vi "Load Suite from Index.vi"(8 "error in (no error)":errorcluster, 11 "Path":path) -> (0 "error out":errorcluster, 3 "LUnit Test Suite out":refnum<class "LUnit Test Suite.lvclass">)   [LabVIEW 2020, in "Test Finder.lvclass"]
uses:
  Test Finder.lvclass
  LUnit Test Suite.lvclass
  C:/git/astemes-lunit/source/Runnable.lvclass
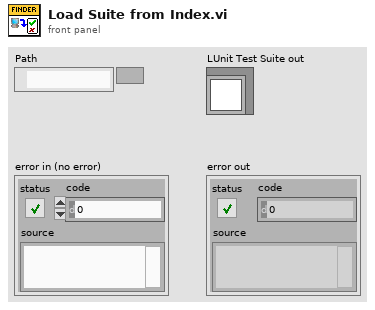
[diagram p1: front panel]
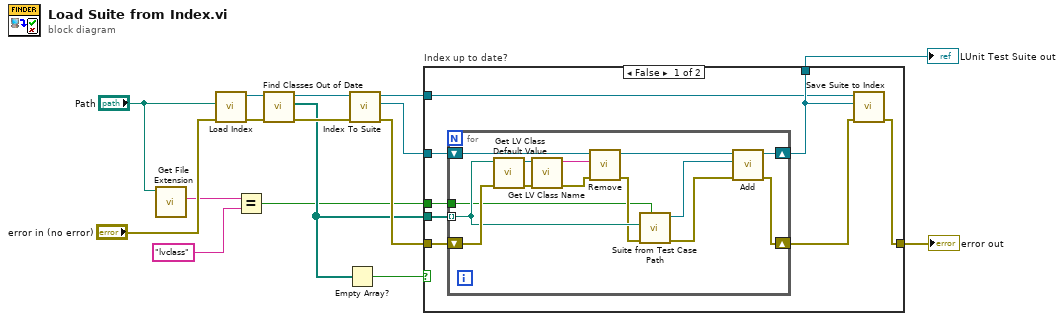
[diagram p0: block diagram]
diagram:
  n1 = call <vilib>:"Get File Extension.vi"("file"="Path") -> ("lowercase file extension"=w3:string)  [unwired: 6 in, 4 out]
  n2 = call "Load Index.vi"("error in (no error)"="error in (no error)", "Path"="Path") -> ("error out"=w9:errorcluster, "Test Finder out"=w8:refnum<class "Test Finder.lvclass">)  [unwired: 8 in]
  n3 = Equal?(x=w3, y="lvclass") -> (x = y?=w1:bool)
  n4 = call "Find Classes Out of Date.vi"("error in (no error)"=w9, "Test Finder In"=w8) -> ("error out"=w11:errorcluster, "Outdated Test Class paths"=w6:path[], "Test Finder Out"=w10:refnum<class "Test Finder.lvclass">)  [unwired: 7 in]
  n5 = Empty Array?(array=w6) -> (empty?=w5:bool)
  n6 = call "Index To Suite.vi"("error in (no error)"=w11, "Test Finder In"=w10) -> ("error out"=w12:errorcluster, "Suite"=w13:refnum<class "LUnit Test Suite.lvclass">, "Test Finder Out"=w14:refnum<class "Test Finder.lvclass">)  [unwired: 7 in]
  n7 = case "Index up to date?" shown="False" w5 {
    tunnel: [w24 w39] -> w16
    tunnel: [w23 w40] -> w15
    tunnel: w14 -> [w21 _]
    tunnel: w13 -> [w20 w40]
    tunnel: w12 -> [w19 w39]
    tunnel: w6 -> [w18 _]
    tunnel: w1 -> [w17 _]
    frame False {
      n8 = for {
        tunnel: w18 -> [w29] mode=indexing
        shift-right: [w37] -> w23
        shift-left: w20 -> [w38]
        shift-right: [w36] -> w22
        shift-left: w19 -> [w31]
        tunnel: w17 -> [w25]
        n9 = call <vilib>:"Get LV Class Default Value.vi"("error in (no error)"=w31, "class path"=w29) -> ("error out"=w34:errorcluster, "object"=w33:refnum<class>)  [unwired: 8 in]
        n10 = call <vilib>:"Get LV Class Name.vi"("error in (no error)"=w34, "object"=w33) -> ("error out"=w30:errorcluster, "class name"=w32:string)  [unwired: 8 in]
        n11 = call "Remove.vi"("error in (no error)"=w30, "Test to Remove"=w32, "LUnit Test Suite In"=w38) -> ("error out"=w28:errorcluster, "LUnit Test Suite Out"=w35:refnum<class "LUnit Test Suite.lvclass">)  [unwired: 7 in]
        n12 = call "Suite from Test Case Path.vi"("Ignore Index?"=w25, "error in (no error)"=w28, "Test Case"=w29) -> ("error out"=w26:errorcluster, "LUnit Test Suite Out"=w27:refnum<class "LUnit Test Suite.lvclass">)  [unwired: 7 in]
        n13 = call "Add.vi"("error in (no error)"=w26, "Runnable"=w27, "LUnit Test Suite In"=w35) -> ("error out"=w36:errorcluster, "LUnit Test Suite Out"=w37:refnum<class "LUnit Test Suite.lvclass">)  [unwired: 7 in]
      }
      n14 = call "Save Suite to Index.vi"("error in (no error)"=w22, "Suite"=w23, "Test Finder In"=w21) -> ("error out"=w24:errorcluster)  [unwired: 8 in]
    }
    frame True {
    }
  }
  "error out" <- w16
  "LUnit Test Suite out" <- w15
